vi "Tension Control.vi"(7 "Output Range":cluster{"output high":dbl, "output low":dbl}[](array[cluster])=[{"output high"=100.0, "output low"=-100.0}] {"output low" format="%.2f"; "output high" format="%.2f"}, 9 "PID gains":T2(array[cluster])=[{"proportional gain (Kc)"=1.0, "integral time (Ti, min)"=0.01, "derivative time (Td, min)"=0.0}] {"derivative time (Td, min)" format="%.3f"; "integral time (Ti, min)" format="%.3f"; "proportional gain (Kc)" format="%.3f"}, 10 "Measured Tension":dbl[](array[numeric]), 11 "Reference Tension":dbl[](array[numeric])) -> (3 "Voltage Output":dbl[](array[numeric]))   [LabVIEW 2021]
uses:
  <vilib>/addons/control/pid/pid.llb/PID (DBL Array).vi
  <vilib>/addons/control/pid/NI_PID_pid.lvlib
panel:
  out "Force Cluster":T1
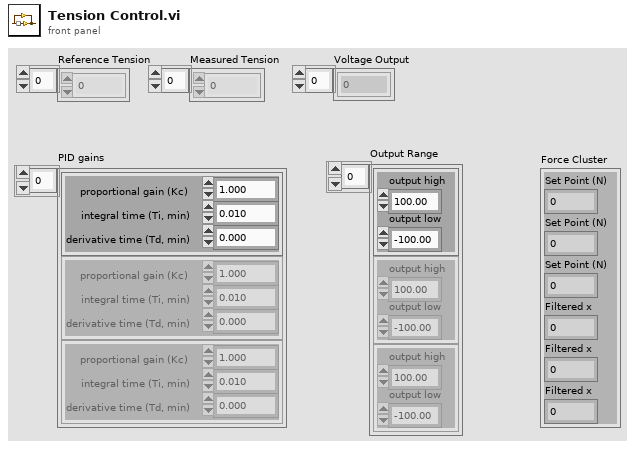
[diagram p1: front panel]
types:
  T1 = cluster{"Set Point (N)":dbl, "Set Point (N)":dbl, "Set Point (N)":dbl, "Filtered x":dbl, "Filtered x":dbl, "Filtered x":dbl}
  T2 = cluster{"proportional gain (Kc)":dbl, "integral time (Ti, min)":dbl, "derivative time (Td, min)":dbl}[]
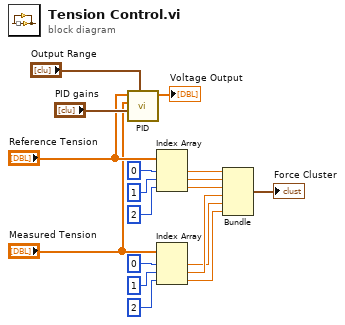
[diagram p0: block diagram]
diagram:
  n1 = call-poly <vilib>:"PID.vi"("output range"="Output Range", "PID gains"="PID gains", "process variable"="Measured Tension", "setpoint"="Reference Tension") -> ("output"=→"Voltage Output":dbl[])  [unwired: 6 in, 1 out]
  n2 = Index Array(array="Reference Tension", index #1=0 ("index"), index #2=1 ("index"), index #3=2 ("index")) -> (element #1=w13:dbl, element #2=w9:dbl, element #3=w6:dbl)
  n3 = Index Array(array="Measured Tension", index #1=0 ("index"), index #2=1 ("index"), index #3=2 ("index")) -> (element #1=w3:dbl, element #2=w4:dbl, element #3=w2:dbl)
  n4 = Bundle("Set Point (N)"=w13, "Set Point (N)"=w9, "Set Point (N)"=w6, "Filtered x"=w4, "Filtered x"=w3, "Filtered x"=w2) -> (→"Force Cluster":T1)  [unwired: 1 in]
